vi "Attached Camera AE.vi"(11 "Camera List in":string[](array[string])=["cam0"]) -> (3 "Camera List out":string[](array[string])=["cam0"])   [LabVIEW 2020]
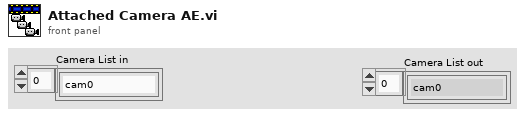
[diagram p1: front panel]
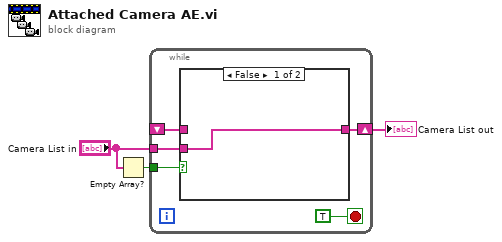
[diagram p0: block diagram]
diagram:
  n1 = Empty Array?(array="Camera List in") -> (empty?=w3:bool)
  n2 = while {
    tunnel: w3 -> [w7]
    shift-right: [w5] -> w1
    shift-left: _ -> [w6]
    tunnel: "Camera List in" -> [w4]
    stop <- TRUE stop-if-true
    n3 = case shown="False" w7 {
      tunnel: w6 -> [_ w10]
      tunnel: [w9 w10] -> w5
      tunnel: w4 -> [w9 _]
      frame False {
      }
      frame True {
      }
    }
  }
  "Camera List out" <- w1
